vi "configure-output.vi"(9 "Current limit":dbl, 10 "Voltage level":dbl, 11 "VISA resource name in":refnum<visa-resource-name>) -> (0 "error out":errorcluster, 3 "VISA resource name out":refnum<visa-resource-name>)   [LabVIEW 2023]
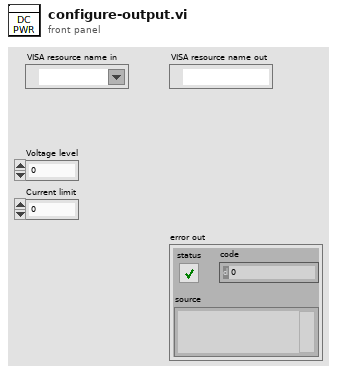
[diagram p1: front panel]
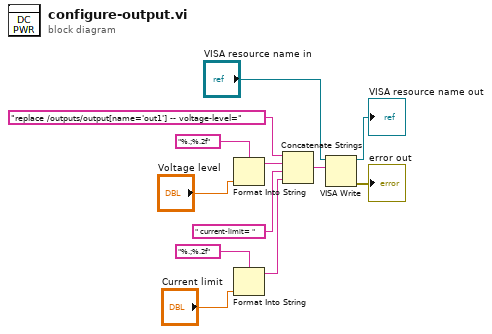
[diagram p0: block diagram]
diagram:
  n1 = Format Into String(format string="%.;%.2f", "Voltage level") -> (resulting string=w10:string)  [unwired: 2 in, 1 out]
  n2 = Format Into String(format string="%.;%.2f", "Current limit") -> (resulting string=w2:string)  [unwired: 2 in, 1 out]
  n3 = Concatenate Strings("replace /outputs/output[name='out1'] -- voltage-level=" ("string"), w10, " current-limit= " ("string"), w2) -> (w12:string)
  n4 = VISA Write(VISA resource name="VISA resource name in", write buffer=w12) -> (VISA resource name out=→"VISA resource name out":refnum<visa-resource-name>, error out=→"error out":errorcluster)  [unwired: 1 in, 1 out]
